vi "FGVLineUpdate.vi"(7 "Enum":T1, 8 "error in":errorcluster, 10 "LineUpdate":u16) -> (0 "error out":errorcluster, 2 "LineUpdate":u16)   [LabVIEW 2016]
uses:
  controls/Enum.ctl
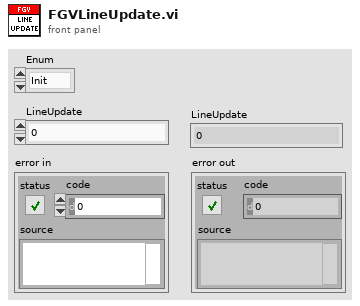
[diagram p1: front panel]
types:
  T1 = typedef "Enum.ctl" = enum16{"Init", "Read", "Write"}
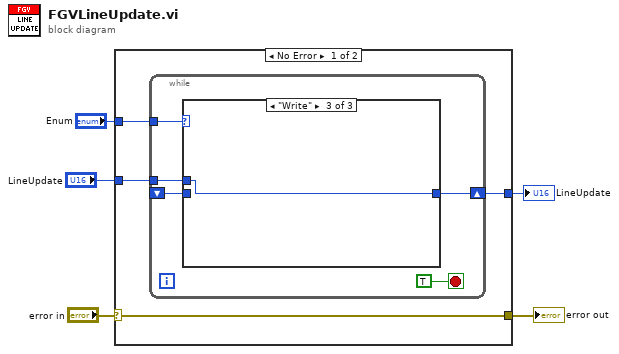
[diagram p0: block diagram]
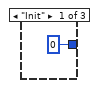
[diagram p2: hidden frame]
diagram:
  n1 = case shown="No Error" "error in" {
    selector: "error in" -> [w8 w19]
    tunnel: "Enum" -> [w9 _]
    tunnel: [w8 w19] -> w4
    tunnel: "LineUpdate" -> [w6 w18]
    tunnel: [w7 w18] -> w1
    frame No Error {
      n2 = while {
        tunnel: w9 -> [w13]
        shift-right: [w11] -> w7
        shift-left: _ -> [w12]
        tunnel: w6 -> [w10]
        stop <- TRUE stop-if-true
        n3 = case shown="\"Write\"" w13 {
          tunnel: w12 -> [_ w16 _]
          tunnel: [u16 0 ("SyncPointIn") w16 w17] -> w11
          tunnel: w10 -> [_ _ w17]
          frame "Init" {
          }
          frame "Read", Default {
          }
          frame "Write" {
          }
        }
      }
    }
    frame Error {
    }
  }
  "error out" <- w4
  "LineUpdate" <- w1
